vi "convert_V_N.vi"(9 "waveform":waveform(dbl), 10 "waveform 2":waveform(dbl)) -> (1 "Array":dbl[](array[numeric]), 2 "Array 2":dbl[](array[numeric]))   [LabVIEW 2014]
panel:
  in  "Boolean":bool
  # "Conversion from the mv/V to the N-m:\n\nThe input straight from the torque transducer is mv/V \n\nBut this is amplified (excited 10V)  \n\nHence the range of votage - torque available: 0-21mv = 0-500 N-m\n\nTo convert the mv/V - N-m we need to look at it UNEXCITED. \n\nIf it is Excited, then the other side  of the equation also needs to be modified. \nIf not, there will be a factor of 10 difference in the equality between them.\n\nHence  the Equation : T = bD + cD^2 , where T is the torque in N-m \n                                                                b =  - 2.7704061E+002 \n                                                                c =    3.36927270E-001\n                                                                                     D =  the deflection measured (mv/V)"
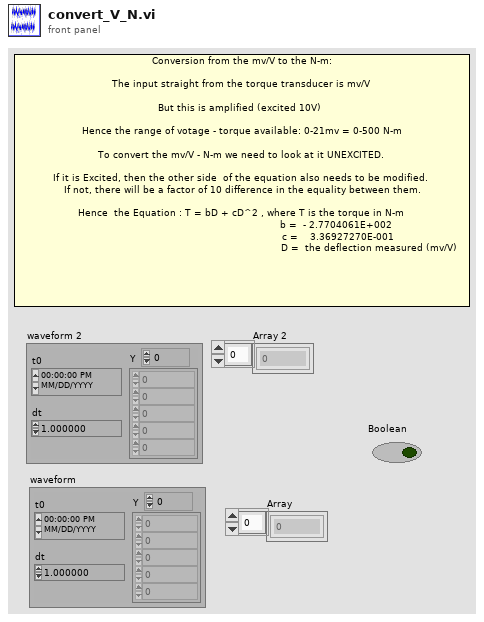
[diagram p1: front panel]
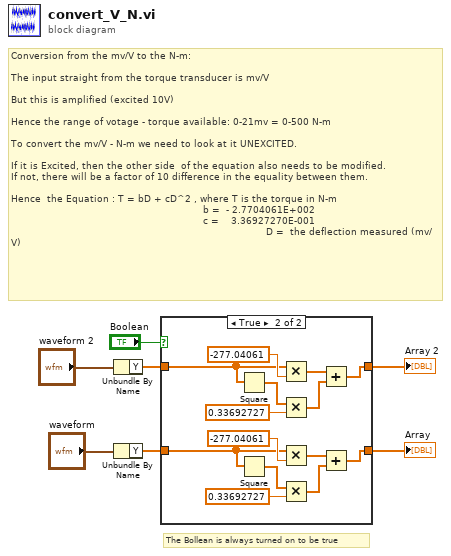
[diagram p0: block diagram]
diagram:
  # "The Bollean is always turned on to be true"
  # "Conversion from the mv/V to the N-m:\n\nThe input straight from the torque transducer is mv/V \n\nBut this is amplified (excited 10V)  \n\nHence the range of votage - torque available: 0-21mv = 0-500 N-m\n\nTo convert the mv/V - N-m we need to look at it UNEXCITED. \n\nIf it is Excited, then the other side  of the equation also needs to be modified. \nIf not, there will be a factor of 10 difference in the equality between them.\n\nHence  the Equation : T = bD + cD^2 , where T is the torque in N-m \n                                                                b =  - 2.7704061E+002 \n                                                                c =    3.36927270E-001\n                                                                                     D =  the deflection measured (mv/V)"
  n1 = Unbundle By Name("waveform 2") -> ("Y"=w3:dbl[])
  n2 = Unbundle By Name("waveform") -> ("Y"=w6:dbl[])
  n3 = case shown="True" "Boolean" {
    tunnel: [w9 w18] -> w2
    tunnel: [w8 w12] -> w1
    tunnel: w6 -> [w9 w10]
    tunnel: w3 -> [w8 w11]
    frame False {
    }
    frame True {
      n4 = Square(x=w11) -> (x^2=w16:dbl[])
      n5 = Square(x=w10) -> (x^2=w22:dbl[])
      n6 = Multiply(x=w11, y=-277.04061) -> (x*y=w14:dbl[])
      n7 = Multiply(x=w16, y=0.33692727) -> (x*y=w13:dbl[])
      n8 = Multiply(x=w10, y=-277.04061) -> (x*y=w20:dbl[])
      n9 = Multiply(x=w22, y=0.33692727) -> (x*y=w19:dbl[])
      n10 = Add(x=w14, y=w13) -> (x+y=w12:dbl[])
      n11 = Add(x=w20, y=w19) -> (x+y=w18:dbl[])
    }
  }
  "Array" <- w2
  "Array 2" <- w1
